vi "libssh2_channel_read.vi"(8 "error in (no error)":errorcluster, 10 "buflen":i64=1024, 11 "channel":T1) -> (0 "error out":errorcluster, 2 "buf":u8[](array[numeric]), 3 "return value":i64)   [LabVIEW 2013, in "libssh2.lvlib"]
doc: "Reads data from the standard I/O substream."
uses:
  libssh2.lvlib
  Channel Refnum.ctl
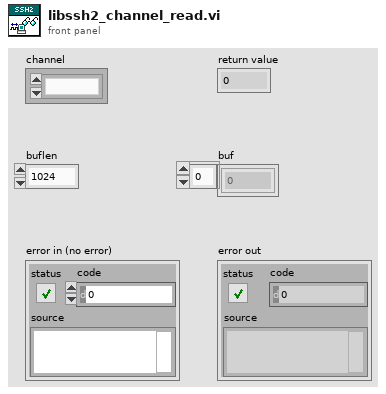
[diagram p1: front panel]
types:
  T1 = typedef "libssh2.lvlib/Channel Refnum.ctl" = refnum<k1>
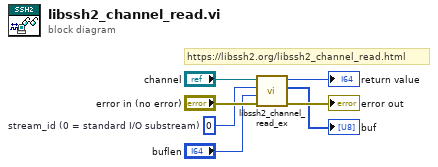
[diagram p0: block diagram]
diagram:
  w1 = 0  # stream_id (0 = standard I/O substream)
  # "https://libssh2.org/libssh2_channel_read.html"
  n1 = call "libssh2_channel_read_ex.vi"("error in (no error)"="error in (no error)", "buflen"="buflen", "stream_id"=w1, "channel"="channel") -> ("error out"=→"error out":errorcluster, "buf"=→"buf":u8[], "return value"=→"return value":i64)  [unwired: 5 in]
